vi "concatenate-array.vi"(11 "Array":string[](array[string])) -> (3 "delimited string":string)   [LabVIEW 2019]
panel:
  out "delimited string 2":string
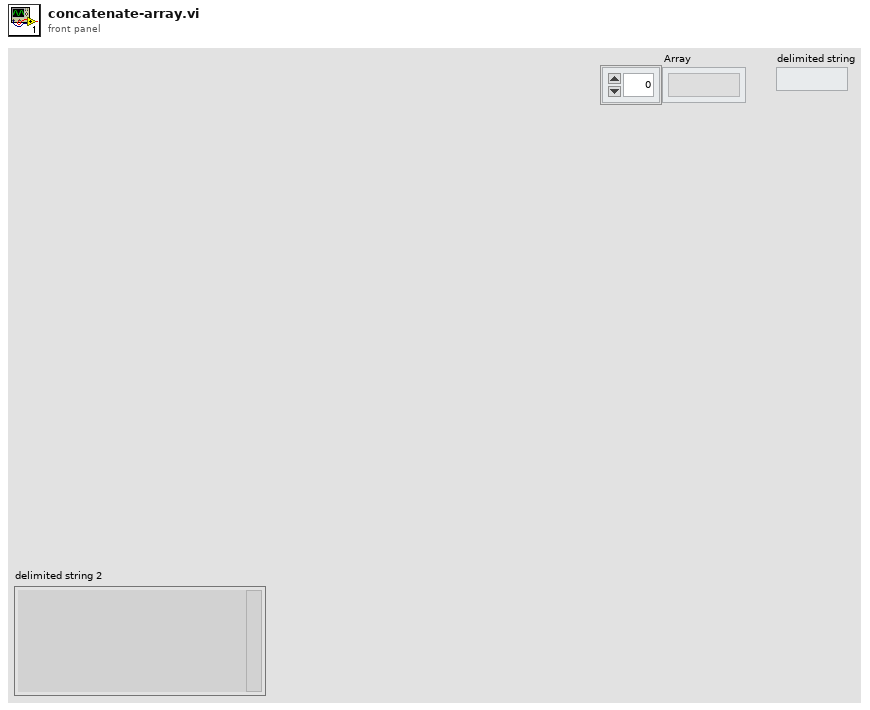
[diagram p1: front panel]
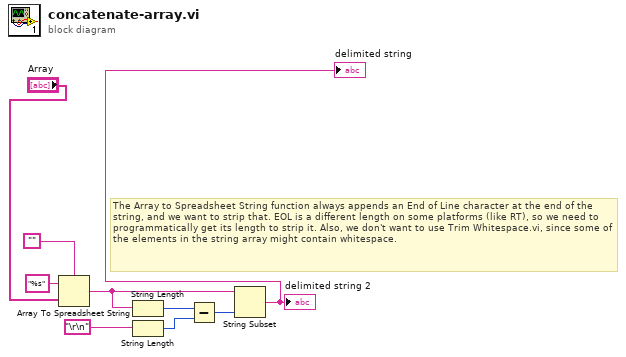
[diagram p0: block diagram]
diagram:
  # "The Array to Spreadsheet String function always appends an End of Line character at the end of the string, and we want to strip that. EOL is a different length on some platforms (like RT), so we need to programmatically get its length to strip it. Also, we don't want to use Trim Whitespace.vi, since some of the elements in the string array might contain whitespace."
  n1 = Array To Spreadsheet String(delimiter (Tab)="", array="Array", 3:"%s" ("format string")) -> (spreadsheet string=w5:string)
  n2 = String Length(string=w5) -> (length=w7:i32)
  n3 = String Length(string="\r\n") -> (length=w6:i32)
  n4 = Subtract(x=w7, y=w6) -> (x-y=w4:i32)
  n5 = String Subset(string=w5, length (rest)=w4) -> (substring=→"delimited string" →"delimited string 2":string)  [unwired: 1 in]
